vi "Immediate Transient Trigger.vi"(8 "error in (no error)":errorcluster {"code" format="%.0x"}, 10 "Channel Name (1)":string="1", 11 "VISA resource name":refnum<visa-resource-name>) -> (0 "error out":errorcluster {"code" format="%.0x"}, 3 "VISA resource name out":refnum<visa-resource-name>)   [LabVIEW 2018, in "Agilent N6700 Series.lvlib"]
doc: "Generates an immediate transient trigger regardless of the selected trigger source. Output triggers affect the following properties: voltage, current, and current limit. You must initiate the output trigger system before you can send any triggers. \n\nWhen sent, the output trigger will:\n(1) Initiate an output change as specified by the Current Triggered or Voltage Triggered.\n(2) Clears the WTG-tran bit in the Status Operation Condition\nregister after the transient trigger sequence has completed."
uses:
  Agilent N6700 Series.lvlib
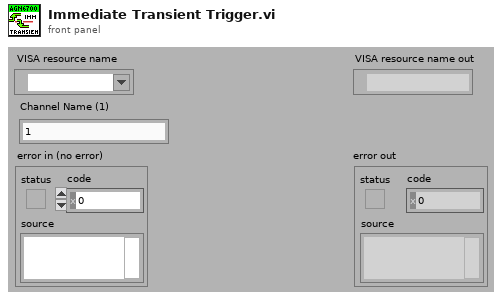
[diagram p1: front panel]
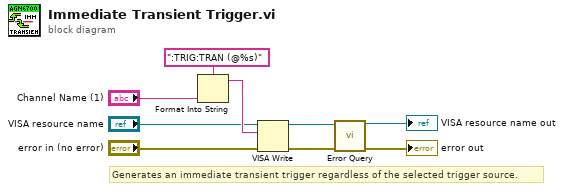
[diagram p0: block diagram]
diagram:
  # "Generates an immediate transient trigger regardless of the selected trigger source."
  n1 = Format Into String(format string=":TRIG:TRAN (@%s)", "Channel Name (1)") -> (resulting string=w9:string)  [unwired: 2 in, 1 out]
  n2 = VISA Write(VISA resource name="VISA resource name", write buffer=w9, error in (no error)="error in (no error)") -> (VISA resource name out=w2:refnum<visa-resource-name>, error out=w1:errorcluster)  [unwired: 1 out]
  n3 = call "Error Query.vi"("VISA resource name"=w2, "error in (no error)"=w1) -> ("VISA resource name out"=→"VISA resource name out":refnum<visa-resource-name>, "error out"=→"error out":errorcluster)  [unwired: 10 in, 2 out]
